vi "PAS.vi"() -> ()   [LabVIEW 2019]
doc: "This example demonstrates how to acquire a continuous amount of data (Waveform) using the DAQ device's internal clock. It also shows how to synchronize two devices for different device families (E Series, S Series, M Series, X Series, DSA, and SC Express), to simultaneously acquire the data.\n\nFor instructions on how to connect your signals to the DAQ device, refer to your device documentation."
uses:
  Program Files/National Instruments/LabVIEW 2019/examples/Instrument IO/Serial/support/Serial - Settings.ctl
  <vilib>/Utility/error.llb/DialogType.ctl
  <vilib>/DAQmx/read.llb/DAQmx Read (Analog 1D Wfm NChan NSamp).vi
  <vilib>/DAQmx/configure/timing.llb/DAQmx Timing (Sample Clock).vi
  <vilib>/DAQmx/configure/trigger.llb/DAQmx Start Trigger (Digital Edge).vi
  <vilib>/DAQmx/miscellaneous.llb/DAQmx Fill In Error Info.vi
  <vilib>/Instr/_visa.llb/VISA Configure Serial Port (Instr).vi
panel:
  in  "Pass Logger":T1(tab)=enum."Noise config"
  out "CO2 chart":waveform(dbl)[](graph)=[{"t0"=timestamp(3652954538.9343734 s since 1904-01-01), "dt"=0.0, "Y"=[597.0], "attributes"=variant("NI_ChannelName"=variant(string "SCD30 CO2"), "NI_UnitDescription"=variant(string "ppm"))}, {"t0"=timestamp(3652954538.9343734 s since 1904-01-01), "dt"=0.0, "Y"=[25.1], "attributes"=variant("NI_ChannelName"=variant(string "SCD30 Temp"), "NI_UnitDescription"=variant(string "C"))}, {"t0"=timestamp(3652954538.9343734 s since 1904-01-01), "dt"=0.0, "Y"=[30.52], "attributes"=variant("NI_ChannelName"=variant(string "SCD30 Humidity"), "NI_UnitDescription"=variant(string "%"))}, {"t0"=timestamp(3652954538.9343734 s since 1904-01-01), "dt"=0.0, "Y"=[23.74], "attributes"=variant("NI_ChannelName"=variant(string "BME680 Temp"), "NI_UnitDescription"=variant(string "C"))}, {"t0"=timestamp(3652954538.9343734 s since 1904-01-01), "dt"=0.0, "Y"=[1014.98], "attributes"=variant("NI_ChannelName"=variant(string "hPa"), "NI_UnitDescription"=variant(string "BME680 Pressure"))}, {"t0"=timestamp(3652954538.9343734 s since 1904-01-01), "dt"=0.0, "Y"=[34.0], "attributes"=variant("NI_ChannelName"=variant(string "BME680 Humidity"), "NI_UnitDescription"=variant(string "%"))}, {"t0"=timestamp(3652954538.9343734 s since 1904-01-01), "dt"=0.0, "Y"=[186.22], "attributes"=variant("NI_ChannelName"=variant(string "BME680 Gas"), "NI_UnitDescription"=variant(string "KOhms"))}]
  in  "Stop":bool
  in  "Enable logging":bool=TRUE caption="Enable"
  in  "File config":T2={"Filepath"=path "C:/Users/Administrator/Desktop/DAQ PAS/Test data", "Test ID"="noise_test", "PC"="69DTQV2"}
  out "Lockin chart":waveform(dbl)[](graph)=[{"t0"=timestamp(3652954539.9158244 s since 1904-01-01), "dt"=1.999, "Y"=[1.7038940113482404], "attributes"=variant("NI_ChannelName"=variant(string "Phase - Mic Diff"), "NI_UnitDescription"=variant(string "Rad"))}, {"t0"=timestamp(3652954539.9158244 s since 1904-01-01), "dt"=1.999, "Y"=[0.00023496982767815845], "attributes"=variant("NI_ChannelName"=variant(string "Amplitude - Mic Diff"), "NI_UnitDescription"=variant(string "Volt"))}]
  out "Lockin output 1":T3={"X"=-1.559084274076101e-05, "Y"=0.00011644582689993115, "R"=0.00011748491383907923, "θ"=1.7038940113482404, "Amp"=0.00023496982767815845, "dt"=1.999, "Active channel"="Mic Diff", "Ref channel"="Heater V"} {"X" format="%#_3g"; "Y" format="%#_3g"; "R" format="%#_3g"}
  out "Reference sesnsor readings":T4={"SCD30 CO2"=597.0, "SCD30 Temp (C)"=25.1, "SCD30 RH (%)"=30.52, "BME680 Temp (C) "=23.74, "BME680 Presssure (hPa)"=1014.98, "BME680 RH (%) "=34.0, "BME680 Gas (KOhms)"=186.22}
  in  "Sampling config":cluster{"Fs":dbl, "#s":dbl}={"Fs"=1000.0, "#s"=2000.0} {"Fs" format="%.2p"}
  in  "Config 1":cluster{"Ref Index":i32, "Active Index":i32}={"Ref Index"=5, "Active Index"=6}
  out "Lockin output 5":T3={"X"=0.37536389386861024, "Y"=0.0013716177488202607, "R"=0.3753663998754473, "θ"=0.0036540851862719523, "Amp"=0.7507327997508946, "dt"=1.999, "Active channel"="Heater V", "Ref channel"="Heater V"} {"X" format="%#_3g"; "Y" format="%#_3g"; "R" format="%#_3g"}
  out "Lockin output 6":T3={"X"=0.1699784370483448, "Y"=0.00018854597623423037, "R"=0.1699785416191799, "θ"=0.0011092342192296652, "Amp"=0.3399570832383598, "dt"=1.999, "Active channel"="Heater Current", "Ref channel"="Heater V"} {"X" format="%#_3g"; "Y" format="%#_3g"; "R" format="%#_3g"}
  out "Lockin output 4":T3={"X"=1.8899040346349075e-15, "Y"=0.0, "R"=1.8899040346349075e-15, "θ"=0.0, "Amp"=3.779808069269815e-15, "dt"=1.999, "Active channel"="Diode Heater", "Ref channel"="Heater V"} {"X" format="%#_3g"; "Y" format="%#_3g"; "R" format="%#_3g"}
  out "Lockin output 3":T3={"X"=-8.538159705352245e-05, "Y"=6.73470760641473e-05, "R"=0.00010874578506682508, "θ"=2.4737323056749747, "Amp"=0.00021749157013365017, "dt"=1.999, "Active channel"="Mic Ref", "Ref channel"="Heater V"} {"X" format="%#_3g"; "Y" format="%#_3g"; "R" format="%#_3g"}
  out "Lockin output 2":T3={"X"=-6.84277126901535e-05, "Y"=-5.017797433685053e-05, "R"=8.485388012669677e-05, "θ"=-2.508866135574671, "Amp"=0.00016970776025339353, "dt"=1.999, "Active channel"="Mic Active", "Ref channel"="Heater V"} {"X" format="%#_3g"; "Y" format="%#_3g"; "R" format="%#_3g"}
  in  "Config 5":cluster{"Ref Index":i32, "Active Index":i32}={"Ref Index"=5, "Active Index"=5}
  in  "Config 4":cluster{"Ref Index":i32, "Active Index":i32}={"Ref Index"=5, "Active Index"=2}
  in  "Config 3":cluster{"Ref Index":i32, "Active Index":i32}={"Ref Index"=5, "Active Index"=1}
  in  "Config 2":cluster{"Ref Index":i32, "Active Index":i32}={"Ref Index"=5, "Active Index"=0}
  in  "Config 6":cluster{"Ref Index":i32, "Active Index":i32}={"Ref Index"=5, "Active Index"=7}
  out "Lockin output 1":T3={"X"=-1.559084274076101e-05, "Y"=0.00011644582689993115, "R"=0.00011748491383907923, "θ"=1.7038940113482404, "Amp"=0.00023496982767815845, "dt"=1.999, "Active channel"="Mic Diff", "Ref channel"="Heater V"} {"X" format="%#_3g"; "Y" format="%#_3g"; "R" format="%#_3g"}
  in  "VISA resource name 2":refnum<visa-resource-name>="COM6"
  in  "Serial Settings":T5={"baud rate"=9600, "data bits"=8, "parity"=enum."None", "stop bits"=10, "flow control"=0} {"flow control" items=["None"=0, "XON/XOFF"=1, "RTS/CTS"=2, "DTR/DSR"=4]; "stop bits" items=["1.0"=10, "1.5"=15, "2.0"=20]; "data bits" min=5 max=8 step=1; "baud rate" items=["75"=75, "110"=110, "134"=134, "150"=150, "300"=300, "600"=600, "1200"=1200, "1800"=1800, "2400"=2400, "4800"=4800, "7200"=7200, "9600"=9600, "14400"=14400, "19200"=19200, "28800"=28800, "38400"=38400, "56000"=56000, "57600"=57600, "115200"=115200, "128000"=128000, "230400"=230400]}
  out "Waveform":waveform(dbl)(graph)={"t0"=timestamp(3652954539.9157805 s since 1904-01-01), "dt"=0.001, "Y"=array[2000 elements], "attributes"=variant("NI_ChannelName"=variant(string "Mic Diff"), "NI_UnitDescription"=variant(string "Volts"))}
  out "Channel names":T6={"Ref channel"="Mic Ref", "Active channel"="Mic Active"}
  in  "Config":T7={"Ref Index"=1, "Active Index"=0, "Gain"=0.984, "Channel name"="Mic Diff", "Enable"=TRUE}
  in  "Waveform config":T8={"Frequency"=70.0, "Voltage"=1.5, "Signal type"=enum."Sine Wave", "Square wave duty cycle (%)"=50.0, "physical channels"="Dev1/ao0", "name to assign"="Heater AO"} {"Square wave duty cycle (%)" format="%0.2f"}
  in  "Vref config":T9={"Voltage"=5.0, "physical channels"="Dev1/ao1", "name to assign"="Diode Vref"}
  out "Channel name":string="Heater Shunt"
  in  "Config":T10={"Channel Index"=4, "Resistance"=1, "Channel name"="Heater Current"}
  out "Microphone Waveform":waveform(dbl)[](graph)=[{"t0"=timestamp(3652954539.915769 s since 1904-01-01), "dt"=0.001, "Y"=array[2000 elements], "attributes"=variant("NI_ChannelName"=variant(string "Mic Active"), "NI_UnitDescription"=variant(string "Volts"))}, {"t0"=timestamp(3652954539.9157805 s since 1904-01-01), "dt"=0.001, "Y"=array[2000 elements], "attributes"=variant("NI_ChannelName"=variant(string "Mic Ref"), "NI_UnitDescription"=variant(string "Volts"))}, {"t0"=timestamp(3652954539.9157915 s since 1904-01-01), "dt"=0.001, "Y"=array[2000 elements], "attributes"=variant("NI_ChannelName"=variant(string "Diode Heater"), "NI_UnitDescription"=variant(string "Volts"))}, {"t0"=timestamp(3652954539.9158025 s since 1904-01-01), "dt"=0.001, "Y"=array[2000 elements], "attributes"=variant("NI_ChannelName"=variant(string "Diode Amb"), "NI_UnitDescription"=variant(string "Volts"))}, {"t0"=timestamp(3652954539.9158134 s since 1904-01-01), "dt"=0.001, "Y"=array[2000 elements], "attributes"=variant("NI_ChannelName"=variant(string "Heater Shunt"), "NI_UnitDescription"=variant(string "Volts"))}, {"t0"=timestamp(3652954539.9158244 s since 1904-01-01), "dt"=0.001, "Y"=array[2000 elements], "attributes"=variant("NI_ChannelName"=variant(string "Heater V"), "NI_UnitDescription"=variant(string "Volts"))}, {"t0"=timestamp(3652954539.9157805 s since 1904-01-01), "dt"=0.001, "Y"=array[2000 elements], "attributes"=variant("NI_ChannelName"=variant(string "Mic Diff"), "NI_UnitDescription"=variant(string "Volts"))}, {"t0"=timestamp(3652954539.9158134 s since 1904-01-01), "dt"=0.001, "Y"=array[2000 elements], "attributes"=variant("NI_ChannelName"=variant(string "Heater Current"), "NI_UnitDescription"=variant(string "mA"))}]
  out "Heater Waveform":waveform(dbl)[](graph)=[{"t0"=timestamp(3652954539.915769 s since 1904-01-01), "dt"=0.001, "Y"=array[2000 elements], "attributes"=variant("NI_ChannelName"=variant(string "Mic Active"), "NI_UnitDescription"=variant(string "Volts"))}, {"t0"=timestamp(3652954539.9157805 s since 1904-01-01), "dt"=0.001, "Y"=array[2000 elements], "attributes"=variant("NI_ChannelName"=variant(string "Mic Ref"), "NI_UnitDescription"=variant(string "Volts"))}, {"t0"=timestamp(3652954539.9157915 s since 1904-01-01), "dt"=0.001, "Y"=array[2000 elements], "attributes"=variant("NI_ChannelName"=variant(string "Diode Heater"), "NI_UnitDescription"=variant(string "Volts"))}, {"t0"=timestamp(3652954539.9158025 s since 1904-01-01), "dt"=0.001, "Y"=array[2000 elements], "attributes"=variant("NI_ChannelName"=variant(string "Diode Amb"), "NI_UnitDescription"=variant(string "Volts"))}, {"t0"=timestamp(3652954539.9158134 s since 1904-01-01), "dt"=0.001, "Y"=array[2000 elements], "attributes"=variant("NI_ChannelName"=variant(string "Heater Shunt"), "NI_UnitDescription"=variant(string "Volts"))}, {"t0"=timestamp(3652954539.9158244 s since 1904-01-01), "dt"=0.001, "Y"=array[2000 elements], "attributes"=variant("NI_ChannelName"=variant(string "Heater V"), "NI_UnitDescription"=variant(string "Volts"))}, {"t0"=timestamp(3652954539.9157805 s since 1904-01-01), "dt"=0.001, "Y"=array[2000 elements], "attributes"=variant("NI_ChannelName"=variant(string "Mic Diff"), "NI_UnitDescription"=variant(string "Volts"))}, {"t0"=timestamp(3652954539.9158134 s since 1904-01-01), "dt"=0.001, "Y"=array[2000 elements], "attributes"=variant("NI_ChannelName"=variant(string "Heater Current"), "NI_UnitDescription"=variant(string "mA"))}]
  in  "Channel 6 config":T11={"Channel"="Dev1/ai5", "Vmax"=2.0, "Vmin"=0.0, "name to assign"="Heater V", "input terminal configuration"=10106} {"input terminal configuration" items=["Default"=-1, "RSE"=10083, "NRSE"=10078, "Differential"=10106, "Pseudodifferential"=12529]; "Vmin" format="%0.2f"; "Vmax" format="%0.2f"}
  in  "Channel 5 config":T11={"Channel"="Dev1/ai4", "Vmax"=0.2, "Vmin"=0.0, "name to assign"="Heater Shunt", "input terminal configuration"=10106} {"input terminal configuration" items=["Default"=-1, "RSE"=10083, "NRSE"=10078, "Differential"=10106, "Pseudodifferential"=12529]; "Vmin" format="%0.2f"; "Vmax" format="%0.2f"}
  in  "Channel 4 config":T11={"Channel"="Dev1/ai3", "Vmax"=1.0, "Vmin"=0.0, "name to assign"="Diode Amb", "input terminal configuration"=10083} {"input terminal configuration" items=["Default"=-1, "RSE"=10083, "NRSE"=10078, "Differential"=10106, "Pseudodifferential"=12529]; "Vmin" format="%0.2f"; "Vmax" format="%0.2f"}
  in  "Channel 3 config":T11={"Channel"="Dev1/ai2", "Vmax"=0.5, "Vmin"=0.0, "name to assign"="Diode Heater", "input terminal configuration"=10083} {"input terminal configuration" items=["Default"=-1, "RSE"=10083, "NRSE"=10078, "Differential"=10106, "Pseudodifferential"=12529]; "Vmin" format="%0.2f"; "Vmax" format="%0.2f"}
  in  "Channel 2 config":T11={"Channel"="Dev1/ai1", "Vmax"=3.0, "Vmin"=-3.0, "name to assign"="Mic Ref", "input terminal configuration"=10083} {"input terminal configuration" items=["Default"=-1, "RSE"=10083, "NRSE"=10078, "Differential"=10106, "Pseudodifferential"=12529]; "Vmin" format="%0.2f"; "Vmax" format="%0.2f"}
  in  "Channel 1 config":T11={"Channel"="Dev1/ai0", "Vmax"=3.0, "Vmin"=-3.0, "name to assign"="Mic Active", "input terminal configuration"=10083} {"input terminal configuration" items=["Default"=-1, "RSE"=10083, "NRSE"=10078, "Differential"=10106, "Pseudodifferential"=12529]; "Vmin" format="%0.2f"; "Vmax" format="%0.2f"}
  # "PAS Logger"
  # "(ppm)"
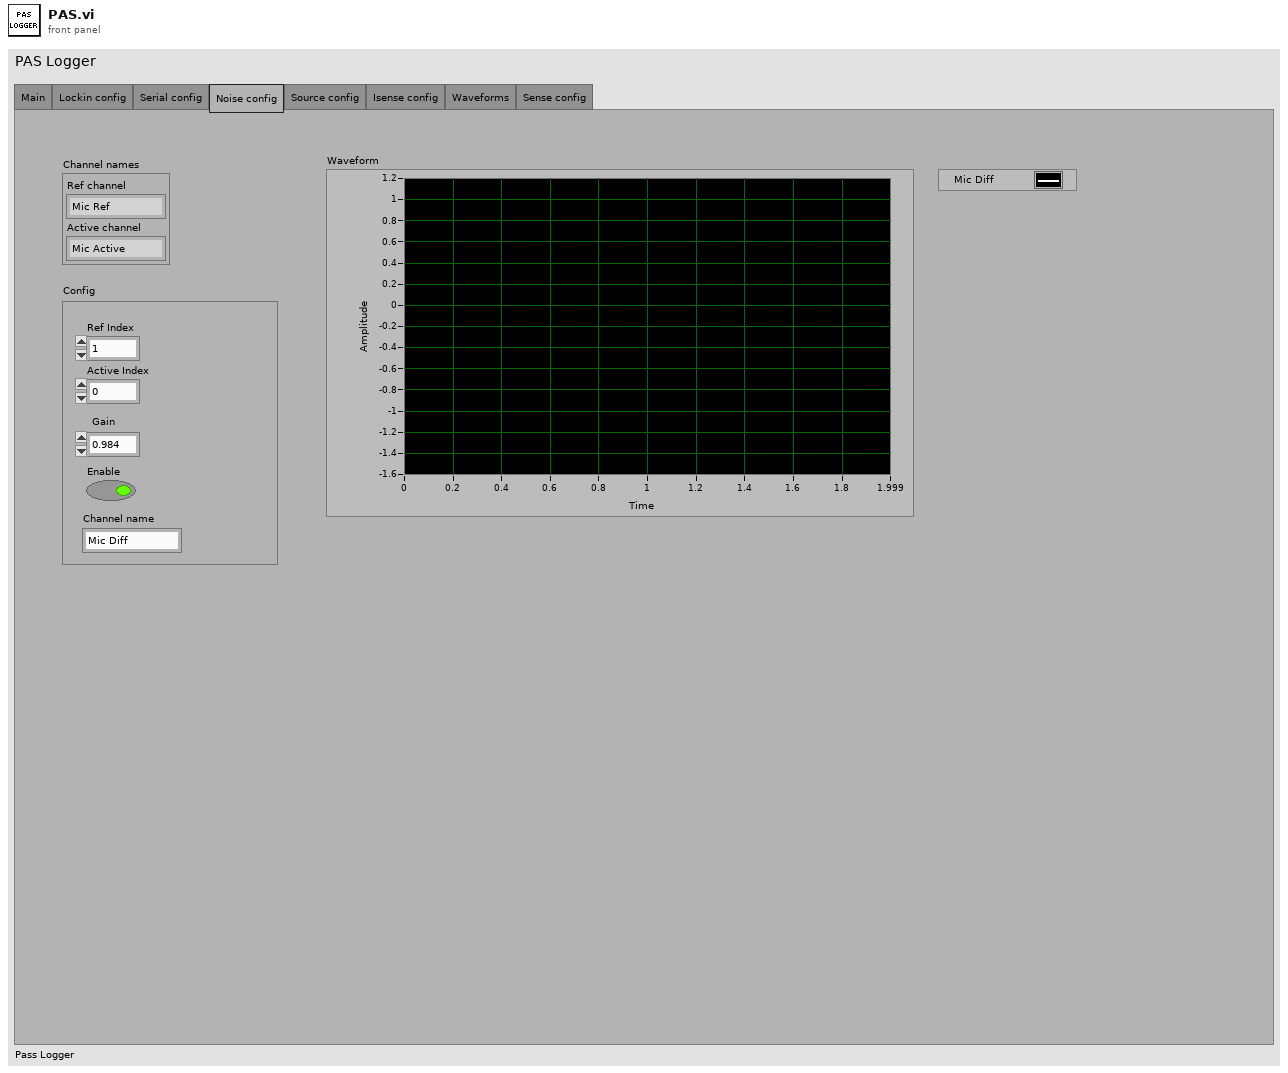
[diagram p1: front panel]
types:
  T1 = enum32{"Main", "Lockin config", "Serial config", "Noise config", "Source config", "Isense config", "Waveforms", "Sense config"}
  T2 = cluster{"Filepath":path, "Test ID":string, "PC":string}
  T3 = cluster{"X":dbl, "Y":dbl, "R":dbl, "θ":dbl, "Amp":dbl, "dt":dbl, "Active channel":string, "Ref channel":string}
  T4 = cluster{"SCD30 CO2":dbl, "SCD30 Temp (C)":dbl, "SCD30 RH (%)":dbl, "BME680 Temp (C) ":dbl, "BME680 Presssure (hPa)":dbl, "BME680 RH (%) ":dbl, "BME680 Gas (KOhms)":dbl}
  T5 = typedef "Serial - Settings.ctl" = cluster{"baud rate":u32, "data bits":u16, "parity":enum16{"None", "Odd", "Even", "Mark", "Space"}, "stop bits":u16, "flow control":u16}
  T6 = cluster{"Ref channel":string, "Active channel":string}
  T7 = cluster{"Ref Index":i32, "Active Index":i32, "Gain":dbl, "Channel name":string, "Enable":bool}
  T8 = cluster{"Frequency":dbl, "Voltage":dbl, "Signal type":enum16{"Sine Wave", "Triangle Wave", "Square Wave", "Sawtooth Wave"}, "Square wave duty cycle (%)":dbl, "physical channels":tag, "name to assign":string}
  T9 = cluster{"Voltage":dbl, "physical channels":tag, "name to assign":string}
  T10 = cluster{"Channel Index":i32, "Resistance":i32, "Channel name":string}
  T11 = cluster{"Channel":tag, "Vmax":dbl, "Vmin":dbl, "name to assign":string, "input terminal configuration":i32}
  T12 = typedef "DialogType.ctl" = u16
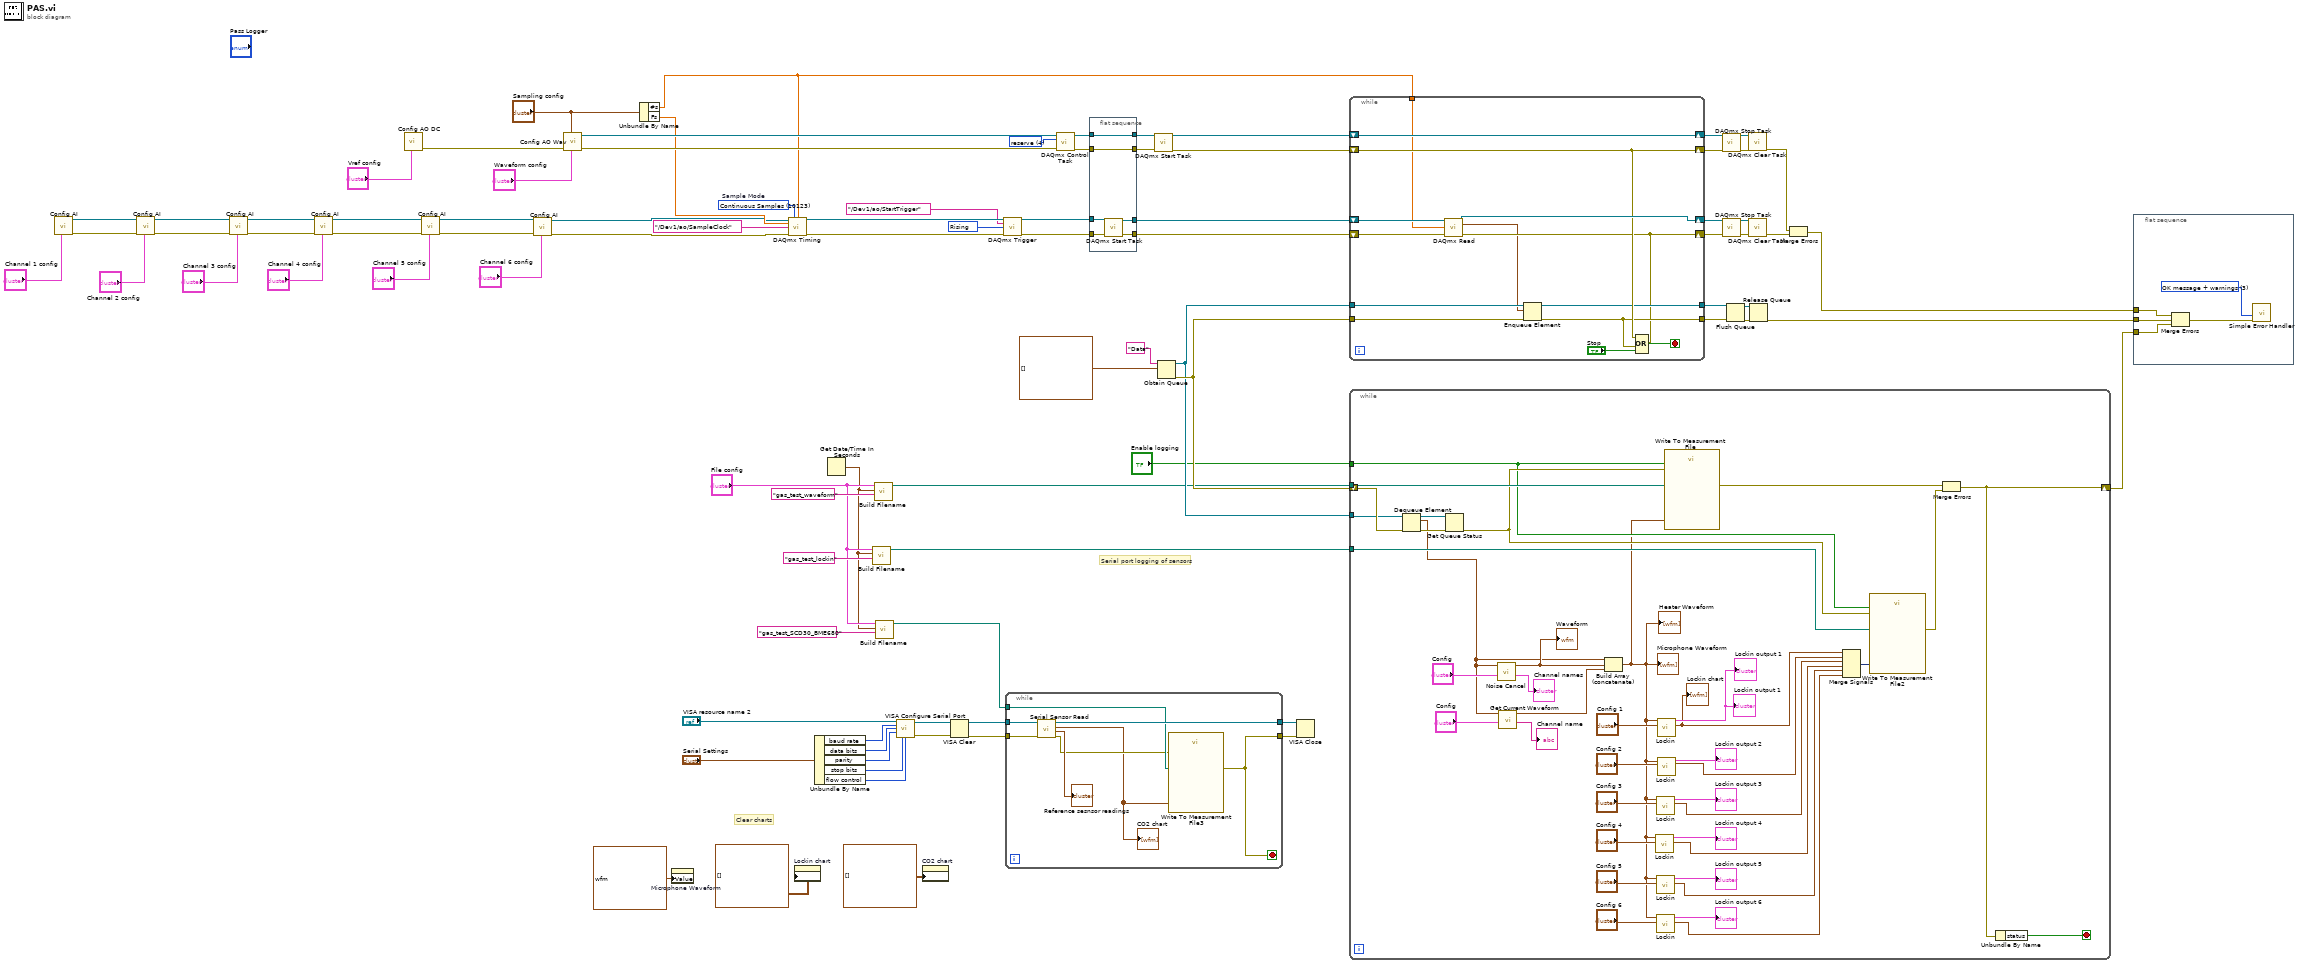
[diagram p0: block diagram]
diagram:
  w71 = 10280 items=["Rising"=10280, "Falling"=10171] ("edge")
  w78 = 4 items=["verify"=2, "reserve"=4, "commit"=3, "unreserve"=5, "abort"=6] ("action")
  w79 = 10123 items=["Finite Samples"=10178, "Continuous Samples"=10123, "Hardware Timed Single Point"=12522]  # Sample Mode
  # "Clear charts"
  # "Serial port logging of sensors"
  n1 = call "Config AI.vi"("Channel config"="Channel 1 config") -> ("error out"=w62:errorcluster, "task out"=w61:refnum<k21>)  [unwired: 9 in]
  n2 = call "Config AI.vi"("Channel config"="Channel 2 config", "error in"=w62, "task in"=w61) -> ("error out"=w43:errorcluster, "task out"=w41:refnum<k21>)  [unwired: 7 in]
  n3 = call "Config AI.vi"("Channel config"="Channel 3 config", "error in"=w43, "task in"=w41) -> ("error out"=w45:errorcluster, "task out"=w44:refnum<k21>)  [unwired: 7 in]
  n4 = call "Config AI.vi"("Channel config"="Channel 4 config", "error in"=w45, "task in"=w44) -> ("error out"=w42:errorcluster, "task out"=w40:refnum<k21>)  [unwired: 7 in]
  n5 = call "Config AO DC.vi"("Channel config"="Vref config") -> ("error out"=w21:errorcluster)  [unwired: 9 in, 1 out]
  n6 = call "Config AI.vi"("Channel config"="Channel 5 config", "error in"=w42, "task in"=w40) -> ("error out"=w39:errorcluster, "task out"=w38:refnum<k21>)  [unwired: 7 in]
  n7 = call "Config AI.vi"("Channel config"="Channel 6 config", "error in"=w39, "task in"=w38) -> ("error out"=w37:errorcluster, "task out"=w36:refnum<k21>)  [unwired: 7 in]
  n8 = call "Config AO Wav.vi"("Channel config"="Waveform config", "Sampling info"="Sampling config", "error in"=w21) -> ("error out"=w60:errorcluster, "task out"=w59:refnum<k21>)  [unwired: 6 in, 1 out]
  n9 = Unbundle By Name("Sampling config") -> ("#s"=w47:dbl, "Fs"=w46:dbl)
  n10 = property on="Microphone Waveform" class="WFGraph (strict)"("Value"=waveform(dbl)[] [{"t0"=timestamp(3651561790.263236 s since 1904-01-01), "dt"=0.001, "Y"=array[2000 elements], "attributes"=variant("NI_ChannelName"=variant(string "Mic Active"), "NI_UnitDescription"=variant(string "Volts"))}, {"t0"=timestamp(3651561790.263247 s since 1904-01-01), "dt"=0.001, "Y"=array[2000 elements], "attributes"=variant("NI_ChannelName"=variant(string "Mic Ref"), "NI_UnitDescription"=variant(string "Volts"))}, {"t0"=timestamp(3651561790.263258 s since 1904-01-01), "dt"=0.001, "Y"=array[2000 elements], "attributes"=variant("NI_ChannelName"=variant(string "Diode Heater"), "NI_UnitDescription"=variant(string "Volts"))}, {"t0"=timestamp(3651561790.263269 s since 1904-01-01), "dt"=0.001, "Y"=array[2000 elements], "attributes"=variant("NI_ChannelName"=variant(string "Diode Amb"), "NI_UnitDescription"=variant(string "Volts"))}, {"t0"=timestamp(3651561790.26328 s since 1904-01-01), "dt"=0.001, "Y"=array[2000 elements], "attributes"=variant("NI_ChannelName"=variant(string "Heater Shunt"), "NI_UnitDescription"=variant(string "Volts"))}, {"t0"=timestamp(3651561790.2632914 s since 1904-01-01), "dt"=0.001, "Y"=array[2000 elements], "attributes"=variant("NI_ChannelName"=variant(string "Heater V"), "NI_UnitDescription"=variant(string "Volts"))}, {"t0"=timestamp(3651561790.263247 s since 1904-01-01), "dt"=0.001, "Y"=array[2000 elements], "attributes"=variant("NI_ChannelName"=variant(string "Mic Diff"), "NI_UnitDescription"=variant(string "Volts"))}, {"t0"=timestamp(3651561790.26328 s since 1904-01-01), "dt"=0.001, "Y"=array[2000 elements], "attributes"=variant("NI_ChannelName"=variant(string "Heater Current"), "NI_UnitDescription"=variant(string "Amps"))}] ("Waveform")) -> ()  [unwired: 2 in, 2 out]
  n11 = call-poly <vilib>:"DAQmx Timing.vi"("task/channels in"=w36, "sample mode"=w79, "samples per channel"=w47, "rate"=w46, "source"=tag "/Dev1/ao/SampleClock", "error in"=w37) -> ("task out"=w72:refnum<k21>, "error out"=w73:errorcluster)  [unwired: 8 in]
  n12 = property on="Lockin chart" class="WFChart (strict)"("History Data"=waveform(dbl)[][] []) -> ()  [unwired: 2 in, 2 out]
  n13 = Unbundle By Name("Serial Settings") -> ("baud rate"=w15:u32, "data bits"=w14:u16, "parity"=w13:enum16{"None", "Odd", "Even", "Mark", "Space"}, "stop bits"=w12:u16, "flow control"=w11:u16)
  n14 = Get Date/Time In Seconds() -> (seconds since 1Jan1904=w18:timestamp)
  n15 = call "Build Filename.vi"("Test type"="gas_test_lockin" ("File Descriptor"), "time stamp"=w18, "File config"="File config") -> ("appended path"=w23:path)  [unwired: 8 in]
  n16 = call "Build Filename.vi"("Test type"="gas_test_waveform" ("File type"), "time stamp"=w18, "File config"="File config") -> ("appended path"=w25:path)  [unwired: 8 in]
  n17 = call "Build Filename.vi"("Test type"="gas_test_SCD30_BME680" ("File Descriptor"), "time stamp"=w18, "File config"="File config") -> ("appended path"=w4:path)  [unwired: 8 in]
  n18 = call-poly "VISA Configure Serial Port"("VISA resource name"="VISA resource name 2", "baud rate (9600)"=w15, "data bits (8)"=w14, "parity (0:none)"=w13, "stop bits (10: 1 bit)"=w12, "flow control (0:none)"=w11) -> ("VISA resource name out"=w9:refnum<visa-resource-name>, "error out"=w10:errorcluster)  [unwired: 3 in, 5 out]
  n19 = property on="CO2 chart" class="WFChart (strict)"("History Data"=waveform(dbl)[][] []) -> ()  [unwired: 2 in, 2 out]
  n20 = VISA Clear(VISA resource name=w9, error in (no error)=w10) -> (VISA resource name out=w8:refnum<visa-resource-name>, error out=w7:errorcluster)
  n21 = call-poly <vilib>:"DAQmx Trigger.vi"("task/channels in"=w72, "source"=tag "/Dev1/ao/StartTrigger", "edge"=w71, "error in"=w73) -> ("task out"=w69:refnum<k21>, "error out"=w70:errorcluster)  [unwired: 10 in]
  n22 = while {
    tunnel: w8 -> [w97]
    tunnel: w7 -> [w96]
    tunnel: [w91] -> w6
    tunnel: [w95] -> w5
    tunnel: w4 -> [w93]
    stop <- w91 stop-if-true
    n23 = call "Serial Sensor Read.vi"("error in (no error)"=w96, "VISA resource name"=w97) -> ("error out"=w92:errorcluster, "Readings"=→"Reference sesnsor readings":T4, "appended array"=w90:waveform(dbl)[], "VISA resource name out"=w95:refnum<visa-resource-name>)  [unwired: 6 in]
    "CO2 chart" <- w90
    n24 = call "Write To Measurement File3"("Signals"=w90, "error in (no error)"=w92, "Filename"=w93) -> ("error out"=w91:errorcluster)  [unwired: 14 in, 2 out]
  }
  n25 = call <vilib>:"DAQmx Control Task.vi"("task/channels in"=w59, "action"=w78, "error in"=w60) -> ("task out"=w68:refnum<k21>, "error out"=w66:errorcluster)  [unwired: 11 in]
  n26 = flat-sequence {
    tunnel: [w103] -> w75
    tunnel: [w102] -> w74
    tunnel: w70 -> [w101]
    tunnel: w69 -> [w100]
    tunnel: w68 -> [w99]
    tunnel: [w99] -> w67
    tunnel: w66 -> [w98]
    tunnel: [w98] -> w65
    frame #0 {
      n27 = call <vilib>:"DAQmx Start Task.vi"("task/channels in"=w100, "error in"=w101) -> ("task out"=w102:refnum<k21>, "error out"=w103:errorcluster)  [unwired: 12 in]
    }
  }
  n28 = call <vilib>:"DAQmx Start Task.vi"("task/channels in"=w67, "error in"=w65) -> ("task out"=w76:refnum<k21>, "error out"=w77:errorcluster)  [unwired: 12 in]
  n29 = Obtain Queue(name (unnamed)="Data" ("名前（名前なし）"), element data type=waveform(dbl)[] [] ("data")) -> (queue out=w50:refnum<queue>, error out=w51:errorcluster)  [unwired: 3 in, 1 out]
  n30 = VISA Close(VISA resource name=w5, error in (no error)=w6) -> ()  [unwired: 1 out]
  n31 = while {
    tunnel: w50 -> [w141]
    shift-right: [w132] -> w49
    shift-left: w51 -> [w142]
    tunnel: w25 -> [w140]
    tunnel: "Enable logging" -> [w136]
    tunnel: w23 -> [w135]
    stop <- w127 stop-if-true
    n32 = Dequeue Element(queue=w141, error in (no error)=w142) -> (queue out=w138:refnum<queue>, element=w126:waveform(dbl)[], error out=w139:errorcluster)  [unwired: 1 in, 1 out]
    n33 = Get Queue Status(queue=w138, error in (no error)=w139) -> (error out=w137:errorcluster)  [unwired: 1 in, 7 out]
    n34 = call "Noise Cancel.vi"("Config"="Config", "array"=w126) -> ("Channel names"=→"Channel names":T6, "waveform out"=w130:waveform(dbl))  [unwired: 8 in]
    "Waveform" <- w130
    n35 = call "Get Current Waveform.vi"("Config"="Config", "array"=w126) -> ("Channel name"=→"Channel name":string, "waveform out"=w125:waveform(dbl))  [unwired: 8 in]
    n36 = Build Array (concatenate)(w126, w130, w125) -> (w104:waveform(dbl)[])
    "Microphone Waveform" <- w104
    "Heater Waveform" <- w104
    n37 = call "Lockin.vi"("Config"="Config 4", "array"=w104) -> ("Output waveform"=w119:waveform(dbl)[], "Lockin output"=→"Lockin output 4":T3)  [unwired: 8 in]
    n38 = call "Lockin.vi"("Config"="Config 3", "array"=w104) -> ("Output waveform"=w120:waveform(dbl)[], "Lockin output"=→"Lockin output 3":T3)  [unwired: 8 in]
    n39 = call "Lockin.vi"("Config"="Config 5", "array"=w104) -> ("Output waveform"=w118:waveform(dbl)[], "Lockin output"=→"Lockin output 5":T3)  [unwired: 8 in]
    n40 = call "Lockin.vi"("Config"="Config 6", "array"=w104) -> ("Output waveform"=w117:waveform(dbl)[], "Lockin output"=→"Lockin output 6":T3)  [unwired: 8 in]
    n41 = call "Lockin.vi"("Config"="Config 1", "array"=w104) -> ("Output waveform"=w105:waveform(dbl)[], "Lockin output"=→"Lockin output 1" →"Lockin output 1":T3)  [unwired: 8 in]
    "Lockin chart" <- w105
    n42 = call "Lockin.vi"("Config"="Config 2", "array"=w104) -> ("Output waveform"=w121:waveform(dbl)[], "Lockin output"=→"Lockin output 2":T3)  [unwired: 8 in]
    n43 = call "Write To Measurement File"("Signals"=w104, "Enable"=w136, "error in (no error)"=w137, "Filename"=w140) -> ("error out"=w133:errorcluster)  [unwired: 13 in, 2 out]
    n44 = Merge Signals(w105, w121, w120, w119, w118, w117) -> (w116:dynamicdata)
    n45 = call "Write To Measurement File2"("Signals"=w116, "Enable"=w136, "error in (no error)"=w137, "Filename"=w135) -> ("error out"=w134:errorcluster)  [unwired: 13 in, 2 out]
    n46 = Merge Errors(w133, w134) -> (w132:errorcluster)
    n47 = Unbundle By Name(w132) -> ("status"=w127:bool)
  }
  n48 = while {
    shift-right: [w152] -> w88
    shift-left: w77 -> [w152]
    shift-right: [w144] -> w84
    shift-left: w75 -> [w154]
    shift-right: [w151] -> w89
    shift-left: w76 -> [w151]
    shift-right: [w153] -> w85
    shift-left: w74 -> [w155]
    tunnel: w47 -> [w150]
    tunnel: [w149] -> w56
    tunnel: [w145] -> w55
    tunnel: w50 -> [w148]
    tunnel: w51 -> [w147]
    stop <- w156 stop-if-true
    n49 = call-poly <vilib>:"DAQmx Read.vi"("task/channels in"=w155, "number of samples per channel"=w150, "error in"=w154) -> ("task out"=w153:refnum<k21>, "data"=w143:waveform(dbl)[], "error out"=w144:errorcluster)  [unwired: 10 in]
    n50 = Enqueue Element(queue=w148, element=w143, error in (no error)=w147) -> (queue out=w149:refnum<queue>, error out=w145:errorcluster)  [unwired: 1 in, 1 out]
    n51 = Compound Arithmetic op=OR(w152, w144, w145, "Stop") -> (w156:bool)
  }
  n52 = call <vilib>:"DAQmx Stop Task.vi"("task/channels in"=w89, "error in"=w88) -> ("task out"=w86:refnum<k21>, "error out"=w87:errorcluster)  [unwired: 12 in]
  n53 = call <vilib>:"DAQmx Stop Task.vi"("task/channels in"=w85, "error in"=w84) -> ("task out"=w82:refnum<k21>, "error out"=w83:errorcluster)  [unwired: 12 in]
  n54 = Flush Queue(queue=w56, error in (no error)=w55) -> (queue out=w57:refnum<queue>, error out=w58:errorcluster)  [unwired: 1 out]
  n55 = call <vilib>:"DAQmx Clear Task.vi"("task in"=w86, "error in"=w87) -> ("error out"=w81:errorcluster)  [unwired: 13 in]
  n56 = call <vilib>:"DAQmx Clear Task.vi"("task in"=w82, "error in"=w83) -> ("error out"=w80:errorcluster)  [unwired: 13 in]
  n57 = Release Queue(queue=w57, error in (no error)=w58) -> (error out=w53:errorcluster)  [unwired: 1 in, 2 out]
  n58 = Merge Errors(w81, w80) -> (w54:errorcluster)
  n59 = flat-sequence {
    tunnel: w54 -> [w161]
    tunnel: w53 -> [w160]
    tunnel: w49 -> [w157]
    frame #0 {
      w159 = T12 3 items=["no dialog", "OK message", "continue or stop message", "OK message + warnings", "continue/stop + warnings"] ("type of dialog (OK msg:1)")
      n60 = Merge Errors(w161, w160, w157) -> (w158:errorcluster)
      n61 = call <vilib>:"Simple Error Handler.vi"("type of dialog (OK msg:1)"=w159, "error in (no error)"=w158) -> ()  [unwired: 3 in, 5 out]
    }
  }
